vi "autosize_listbox_columns.vi"(4 "error in (no error)":errorcluster, 7 "Table Ref":refnum<vi>) -> (0 "error out":errorcluster, 3 "column_widths":i16[](array[numeric]))   [LabVIEW 2020]
doc: "This VI resizes each column of the table specified by Table Ref based on the widest entry of the column. Additionally, if Resize Table? is TRUE, the VI will set the table width based on the number of populated columns."
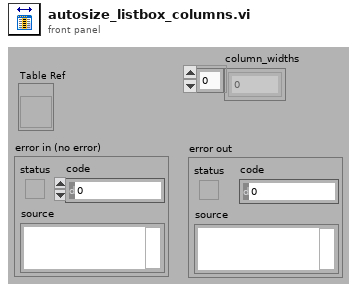
[diagram p1: front panel]
types:
  T1 = enum16{"User-specified Font", "Application Font", "System Font", "Dialog Font"}
  T2 = cluster{"Font Name:":string, "Size":i16, "Strikeout?":bool, "Italic?":bool, "Underline?":bool, "Outline?":bool, "Shadow?":bool, "Bold?":bool}
  T3 = cluster{"left":i16, "top":i16, "right":i16, "bottom":i16}
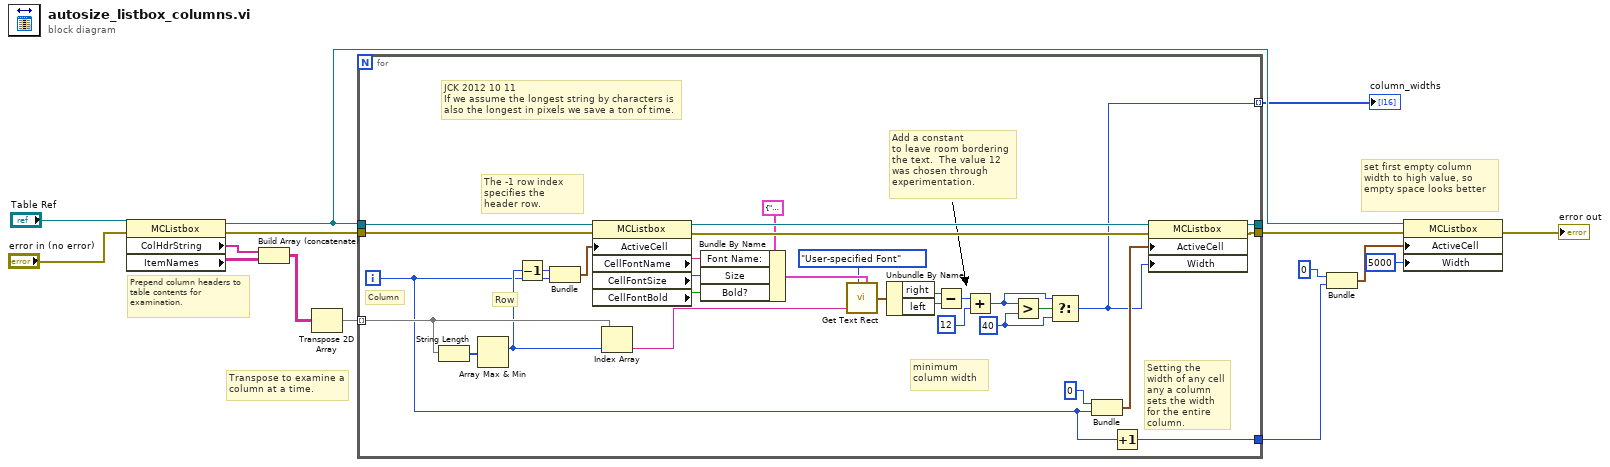
[diagram p0: block diagram]
diagram:
  # "set first empty column width to high value, so empty space looks better"
  # "Prepend column headers to table contents for examination."
  # "Transpose to examine a column at a time."
  n1 = property class="MCListbox"(reference="Table Ref", error in="error in (no error)") -> (reference out=w2:refnum<vi>, error out=w12:errorcluster, "ColHdrString"=w15:string[], "ItemNames"=w11:string[][])
  n2 = Build Array (concatenate)(w15, w11) -> (w14:string[][])
  n3 = Transpose 2D Array(2D array=w14) -> (transposed array=w13:string[][])
  n4 = for {
    tunnel: w13 -> [w46] mode=indexing
    tunnel: w2 -> [w45]
    tunnel: w12 -> [w44]
    tunnel: [w39] -> w7
    tunnel: [w19] -> _
    tunnel: [w17] -> w4
    tunnel: [w16] -> w1 mode=indexing
    i -> [w18]
    w21 = i16 40 ("y")
    # "minimum\ncolumn width"
    # "JCK 2012 10 11\nIf we assume the longest string by characters is also the longest in pixels we save a ton of time."
    # "The -1 row index specifies the header row."
    # "Add a constant\nto leave room bordering the text.  The value 12 was chosen through experimentation."
    # "Row"
    # "Setting the width of any cell any a column sets the width for the entire column."
    # "Column"
    n5 = String Length(string=w46) -> (length=w38:i32[])
    n6 = Array Max & Min(array=w38) -> (max index (indices)=w24:i32)  [unwired: 3 out]
    n7 = Decrement(x=w24) -> (x-1=w34:i32)
    n8 = Bundle(w34, w18) -> (w25:cluster{i32, i32})  [unwired: 1 in]
    n9 = property class="MCListbox"(reference=w45, error in=w44, "ActiveCell"=w25) -> (reference out=w43:refnum<vi>, error out=w42:errorcluster, "CellFontName"=w27:string, "CellFontSize"=w36:u32, "CellFontBold"=w28:bool)
    n10 = Index Array(array=w46, index=w24) -> (element=w23:string)
    n11 = Bundle By Name(cluster=T2 {"Font Name:"="", "Size"=0, "Strikeout?"=FALSE, "Italic?"=FALSE, "Underline?"=FALSE, "Outline?"=FALSE, "Shadow?"=FALSE, "Bold?"=FALSE} ("[user-specified font]"), "Font Name:"=w27, "Size"=w36, "Bold?"=w28) -> (w30:T2)
    n12 = call <vilib>:"Get Text Rect.vi"("desired font(Application)"=T1."User-specified Font", "text"=w23, "[user-specified font]"=w30) -> ("rect"=w31:T3)  [unwired: 6 in]
    n13 = Unbundle By Name(w31) -> ("right"=w32:i16, "left"=w33:i16)
    n14 = Subtract(x=w32, y=w33) -> (x-y=w35:i16)
    n15 = Add(x=w35, y=i16 12) -> (x+y=w20:i16)
    n16 = Greater?(x=w20, y=w21) -> (0:w22:bool)
    n17 = Select(t=w20, s=w22, f=w21) -> (s? t:f=w16:i16)
    n18 = Bundle(0, w18) -> (w40:cluster{i32, i32})  [unwired: 1 in]
    n19 = Increment(x=w18) -> (x+1=w17:i32)
    n20 = property class="MCListbox"(reference=w43, error in=w42, "ActiveCell"=w40, "Width"=w16) -> (reference out=w19:refnum<vi>, error out=w39:errorcluster)
  }
  "column_widths" <- w1
  n21 = Bundle(0, w4) -> (w3:cluster{i32, i32})  [unwired: 1 in]
  n22 = property class="MCListbox"(reference=w2, error in=w7, "ActiveCell"=w3, "Width"=u32 5000 ("Active Cell:Cell Size:Width")) -> (error out=→"error out":errorcluster)  [unwired: 1 out]
